vi "限幅器（I8）.vi"(3 "下限":i8, 4 "X_in":i8, 5 "上限":i8) -> (1 "X_Out":i8)   [LabVIEW 2012]
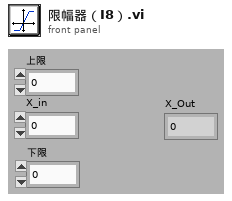
[diagram p1: front panel]
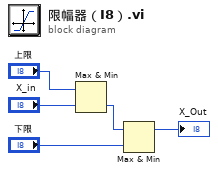
[diagram p0: block diagram]
diagram:
  n1 = Max & Min(x="上限", y="X_in") -> (min(x,y)=w3:i8)  [unwired: 1 out]
  n2 = Max & Min(x=w3, y="下限") -> (max(x,y)=→"X_Out":i8)  [unwired: 1 out]
